vi "Load_Traverse_file.vi"(0 "Setup filename":path) -> (3 "Setup filename Out":path, 4 "Jump Bad Positions":bool, 5 "Table":T2[](array[typedef]) {"Row Duration (mins)" format="%#.1f"; "Row No" min=0; "Trace Gas Concentration (%)" min=0.0 format="%#.2f"; "Emission Rate (l/min)" format="%#.2f"; "Tunnel Speed" format="%#.2f"; "Start X" format="%#.2f"; "Start Y" format="%#.2f"; "Start Z" format="%#.2f"; "End X" format="%#.2f"; "End Y" format="%#.2f"; "End Z" format="%#.2f"; "Averaging time (min)" min=0.0 format="%#.1f"}, 6 "Work in Tunnel Coordinates?":T1)   [LabVIEW 2010]
uses:
  Traverse_cluster.ctl
  Spacing.ctl
  Controls/Multi_run_mode.ctl
  Controls/Tunnel_Coordinates.ctl
panel:
  # "HD:Users"
  # "HD:Users"
  # "X           Y            Z"
  # "Start"
  # "End"
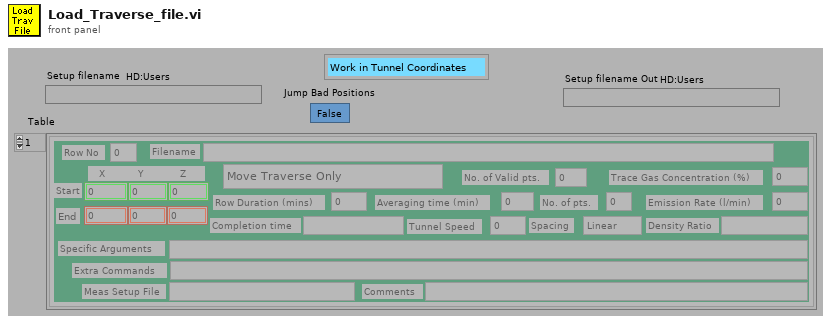
[diagram p1: front panel]
types:
  T1 = typedef "Tunnel_Coordinates.ctl" = enum16{"Work in Tunnel Coordinates", "Work in Model Coordinates"}
  T2 = typedef "Traverse_cluster.ctl" = cluster{"Start X":dbl, "Start Y":dbl, "Start Z":dbl, "End X":dbl, "End Y":dbl, "End Z":dbl, "No. of pts.":i32, "Spacing":T3, "Filename":path, "Tunnel Speed":dbl, "Averaging time (min)":dbl, "Extra Commands":string, "Specific Arguments":string, "Emission Rate (l/min)":dbl, "Trace Gas Concentration (%)":dbl, "Density Ratio":string, "Comments":string, "Row No":i32, "Row Type Selector":T4, "Completion time":string, "Row Duration (mins)":dbl, "No. of Valid pts.":i32, "Meas Setup File":string}
  T3 = typedef "Spacing.ctl" = enum16{"Linear", "Log", "Gauss", "Specified", "N/A"}
  T4 = typedef "Multi_run_mode.ctl" = enum16{"Move Traverse Only", "Set Tunnel Speed Only", "Set Source Only", "Set Measurement Conditions", "Single Measurement", "Vertical Profile", "Lateral Profile", "Longitudinal Profile", "Explore Volume", "Multi-Axis Profile", "Auto Calibrate", "Meas Fast FID Bkgnd", "Check Beam Power", "Scanning Valve Measurement", "Run VI Named:", "Set ADAM Ch", "Wait (minutes)", "Send Message", "Synchronize With:", "Fall Back to this Row", "Turn Off Row Repeating", "Blank Row"}
  T5 = enum16{"All Channel Names", "Valid Channel Names"}
  T6 = enum32{"existing file", "new file", "new or existing file", "existing dir", "new dir", "new or existing dir", "existing file (use LLBs)", "new file (use LLBs)", "new or existing file (use LLBs)", "new or existing file or directory (use LLBs)"}
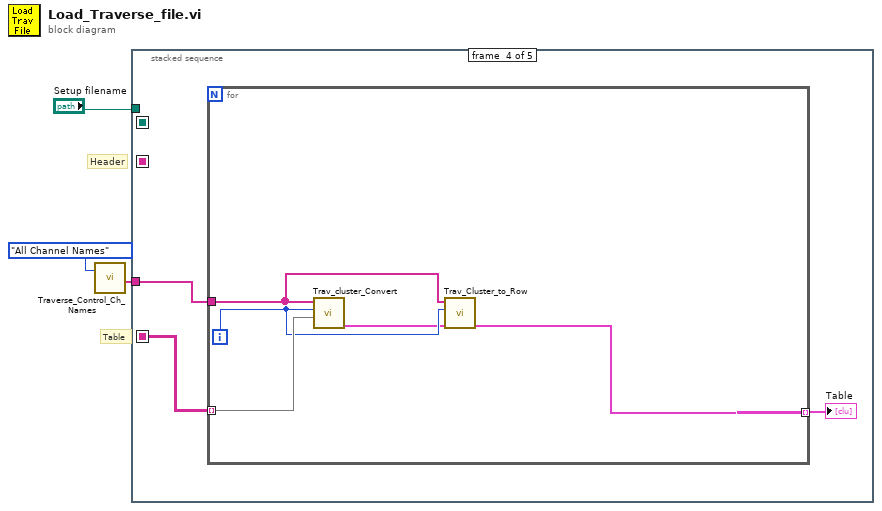
[diagram p0: block diagram]
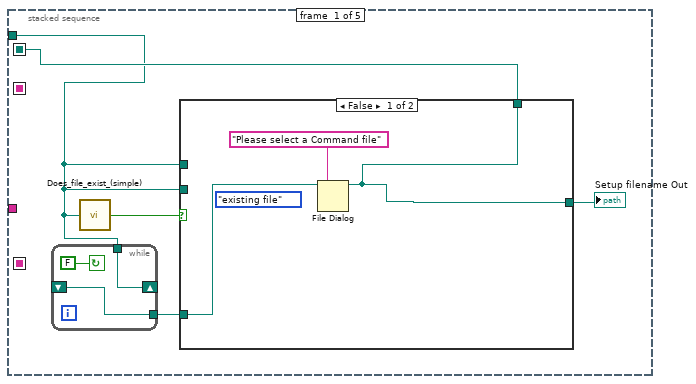
[diagram p2: hidden frame]
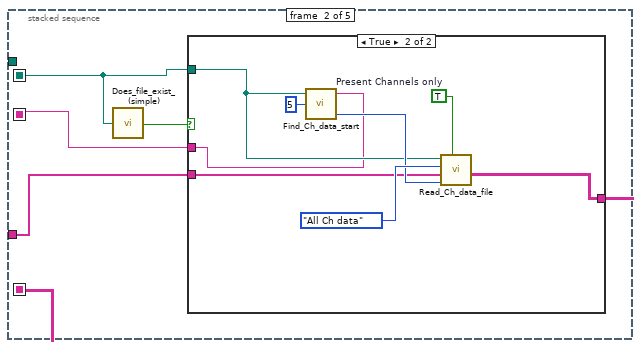
[diagram p4: hidden frame]
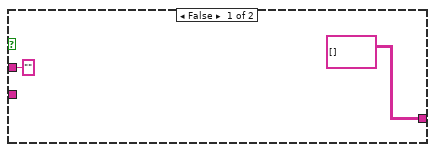
[diagram p5: hidden frame]
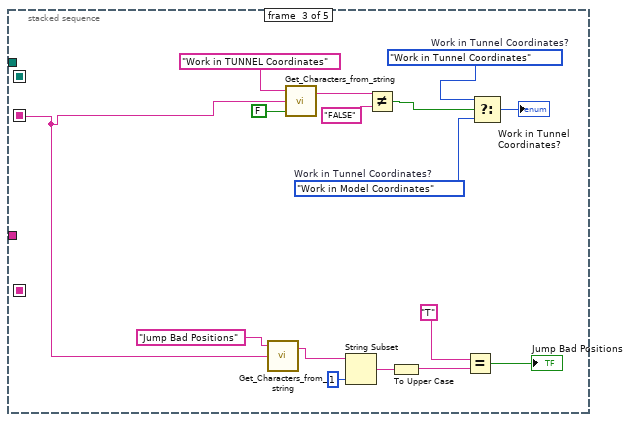
[diagram p6: hidden frame]
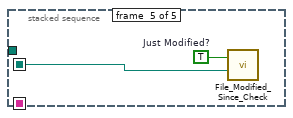
[diagram p7: hidden frame]
diagram:
  # "Header"
  # "Table"
  n1 = call "Traverse_Control_Ch_Names.vi"("Mode"=T5."All Channel Names") -> ("Channel names"=w2:string[])  [unwired: 1 in]
  n2 = stacked-sequence {
    seq-local: [_ w21 _ _ _] -> [_ _ _ w50 _]
    seq-local: [_ w20 _ _ _] -> [_ _ w38 _ _]
    seq-local: [w8 _ _ _ _] -> [_ w18 _ _ w56]
    tunnel: "Setup filename" -> [w4 _ _ _ _]
    tunnel: w2 -> [_ w17 _ w49 _]
    frame #0 {
      n3 = while {
        tunnel: [w10] -> w5
        tunnel: w4 -> [w11]
        shift-left: _ -> [w10]
        shift-right: [w11] -> _
        stop <- FALSE continue-if-true
      }
      n4 = call "Does_file_exist_(simple).vi"("Pathname"=w4) -> ("exists?"=w6:bool)
      n5 = case shown="False" w6 {
        tunnel: w4 -> [_ w16]
        tunnel: [w12 w16] -> w8
        tunnel: [w12 w15] -> w7
        tunnel: w4 -> [_ w15]
        tunnel: w5 -> [w13 _]
        frame False {
          (unwired) T6."existing file" ("select mode (2)")
          n6 = File Dialog(7:"Please select a Command file" ("prompt"), 11:w13) -> (3:w12:path)  [unwired: 1 in, 7 out]
        }
        frame True {
        }
      }
      "Setup filename Out" <- w7
    }
    frame #1 {
      n7 = call "Does_file_exist_(simple).vi"("Pathname"=w18) -> ("exists?"=w19:bool)
      n8 = case shown="True" w19 {
        tunnel: [string[][] [] w26] -> w21
        tunnel: ["" ("character string") w27] -> w20
        tunnel: w18 -> [_ w28]
        tunnel: w17 -> [_ w25]
        frame False {
        }
        frame True {
          w31 = TRUE  # Present Channels only
          n9 = call "Find_Ch_data_start.vi"("Approx No Of Columns"=5, "Filename"=w28) -> ("Start of read offset output"=w29:i32, "String before data"=w27:string)  [unwired: 1 in, 1 out]
          n10 = call "Read_Ch_data_file.vi"("Present Channels only"=w31, "Start of read offset (chars.: 0)"=w29, "Present Channels"=w25, "Output"=enum16{"All Ch data", "The last few rows"}."All Ch data", "Filename"=w28) -> ("Channel Values"=w26:string[][])  [unwired: 4 out]
        }
      }
    }
    frame #2 {
      w41 = Tunnel_Coordinates."Work in Model Coordinates"  # Work in Tunnel Coordinates?
      w43 = Tunnel_Coordinates."Work in Tunnel Coordinates"  # Work in Tunnel Coordinates?
      n11 = call "Get_Characters_from_string.vi"("Input string"=w38, "Variable name"="Jump Bad Positions" ("Label for characters")) -> ("Value"=w33:string)  [unwired: 1 in, 1 out]
      n12 = call "Get_Characters_from_string.vi"("Show Dialog?"=FALSE, "Input string"=w38, "Variable name"="Work in TUNNEL Coordinates" ("Label for characters")) -> ("Value"=w46:string)  [unwired: 1 out]
      n13 = String Subset(string=w33, length (rest)=1 ("length")) -> (substring=w35:string)  [unwired: 1 out]
      n14 = Not Equal?(x=w46, y="FALSE") -> (x != y?=w44:bool)
      n15 = To Upper Case(1:w35) -> (0:w34:string)
      n16 = Equal?(x="T", y=w34) -> (x = y?=→"Jump Bad Positions":bool)
      n17 = Select(t=w43, s=w44, f=w41) -> (s? t:f=→"Work in Tunnel Coordinates?":T1)
    }
    frame #3 {
      n18 = for {
        tunnel: w50 -> [w55] mode=indexing
        tunnel: [w52] -> w48 mode=indexing
        tunnel: w49 -> [w54]
        i -> [w53]
        n19 = call "Trav_cluster_Convert.vi"("Channel Values In"=w55, "Row Number"=w53, "Channel names"=w54) -> ("Traverse line Out"=w51:T2)  [unwired: 1 in, 3 out]
        n20 = call "Trav_Cluster_to_Row.vi"("Traverse line in"=w51, "Row Number"=w53, "Channel names"=w54) -> ("Traverse line Out"=w52:T2)  [unwired: 4 out]
      }
      "Table" <- w48
    }
    frame #4 {
      w57 = TRUE  # Just Modified?
      n21 = call "File_Modified_Since_Check.vi"("Pathname"=w56, "Just Modified?"=w57) -> ()  [unwired: 1 out]
    }
  }
